vi "Teleop.vi"(10 "Match Info":T1={"Autonomous Elapsed Seconds"=0.0, "TeleOp Elapsed Seconds"=0.0, "Disabled Elapsed Seconds"=0.0, "Visited Autonomous"=FALSE, "Visited TeleOp"=FALSE, "Visited Disabled"=FALSE, "Autonomous Settings"={"Autonomous Style"=enum."Independent", "VI Refnum"=refnum}}, 11 "Call Context":T2) -> ()   [LabVIEW 2015]
doc: "This VI is called for each TeleOp packet received from the DS where the robot is not disabled. It is often used to read from the joysticks and update I/O or to update setpoints for timed control loops. It should complete and return within 20 milliseconds or it may miss DS packets."
uses:
  <vilib>/Rock Robotics/WPI/DriverStation/WPI_DriverStationDerivedRobotMode.ctl
  <vilib>/Rock Robotics/WPI/DriverStation/WPI_DriverStationMatch Info.ctl
  <vilib>/Rock Robotics/WPI/Utilities/WPI_GetSetVariantRefNum.vi
  <vilib>/Rock Robotics/Network Tables/NT Write Boolean Array.vi
  <vilib>/Rock Robotics/Network Tables/NT Write Numeric Array.vi
  <vilib>/Rock Robotics/Network Tables/NT Read Boolean.vi
  <vilib>/Rock Robotics/Network Tables/NT Read Number.vi
  <vilib>/Rock Robotics/WPI/RobotDrive/WPI_RobotDriveArcadeDrive_Standard(NoSaturation).vi
panel:
  out "Sample Slider 0":dbl(slide) scale=0.0..5.0
  out "Sample Boolean 1":bool
  out "Sample Boolean 0":bool
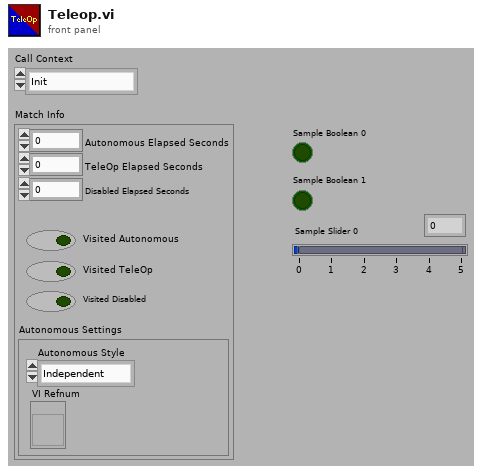
[diagram p1: front panel]
types:
  T1 = typedef "WPI_DriverStationMatch Info.ctl" = cluster{"Autonomous Elapsed Seconds":dbl, "TeleOp Elapsed Seconds":dbl, "Disabled Elapsed Seconds":dbl, "Visited Autonomous":bool, "Visited TeleOp":bool, "Visited Disabled":bool, "Autonomous Settings":cluster{"Autonomous Style":enum16{"Iterative", "Independent"}, "VI Refnum":refnum<vi>}}
  T2 = typedef "WPI_DriverStationDerivedRobotMode.ctl" = enum16{"Init", "Execute", "Stop"}
  T3 = typedef "WPI_CompressorDevRef.ctl" = cluster{"DevStatus":errorcluster, "Pneumatics Control Module":u8}
  T4 = typedef "WPI_JoystickDevRef.ctl" = cluster{"Device":T5}
  T5 = typedef "WPI_JoystickDeviceEnum.ctl" = enum16{"USB 0", "USB 1", "USB 2", "USB 3", "USB 4", "USB 5"}
  T6 = cluster{"Buttons[0]":bool, "Buttons[1]":bool, "Buttons[2]":bool, "Buttons[3]":bool, "Buttons[4]":bool, "Buttons[5]":bool, "Buttons[6]":bool, "Buttons[7]":bool, "Buttons[8]":bool}
  T7 = cluster{"Axes[0]":dbl, "Axes[1]":dbl, "Axes[2]":dbl, "Axes[3]":dbl, "Axes[4]":dbl, "Axes[5]":dbl, "Axes[6]":dbl, "Axes[7]":dbl, "Axes[8]":dbl}
  T8 = typedef "WPI_RobotDriveDevRef.ctl" = cluster{"DevStatus":errorcluster, "Motors[]":T9[], "Square Inputs":bool, "Max Output":dbl}
  T9 = typedef "WPI_MotorControlDeviceRef.ctl" = cluster{"DeviceStatus":errorcluster, "Type":T10, "PWM":cluster{"PWM Channel":T11, "DeadBand":T12}, "CAN":cluster{"Device Number":u8, "Control Mode":T13, "Semaphore":T14, "Max Vout":dbl, "TalonSRX Control Mode":T15}, "Invert":bool}
  T10 = typedef "WPI_MotorControlType.ctl" = enum16{"PWM", "CAN", "CANTalonSRX"}
  T11 = typedef "FPGA_DIOPWMChannel.ctl" = enum8{"PWM 0", "PWM 1", "PWM 2", "PWM 3", "PWM 4", "PWM 5", "PWM 6", "PWM 7", "PWM 8", "PWM 9", "PWM MXP 0", "PWM MXP 1", "PWM MXP 2", "PWM MXP 3", "PWM MXP 4", "PWM MXP 5", "PWM MXP 6", "PWM MXP 7", "PWM MXP 8", "PWM MXP 9", "Invalid"}
  T12 = typedef "WPI_PWMDeadband.ctl" = cluster{"Name":string, "maxPositivePwm":i32, "minPositivePwm":i32, "centerPwm":i32, "maxNegativePwm":i32, "minNegativePwm":i32, "angularRange":u16}
  T13 = typedef "WPI_CANJaguar_ControlMode.ctl" = enum8{"Percent VBus", "Current", "Speed", "Position", "Voltage"}
  T14 = typedef "Semaphore RefNum" = refnum<k1>
  T15 = typedef "WPI_CANTalonSRX_APIControlMode.ctl" = enum8{"Percent VBus", "Speed", "Position", "Slave", "Unchanged / Invalid", "Voltage Compensation", "Current", "Motion Profile"}
  T16 = typedef "WPI_DigitalInputDevRef.ctl" = cluster{"DevStatus":errorcluster, "DIO Channel":T17}
  T17 = typedef "FPGA_DIOChannel.ctl" = enum8{"DIO 0", "DIO 1", "DIO 2", "DIO 3", "DIO 4", "DIO 5", "DIO 6", "DIO 7", "DIO 8", "DIO 9", "DIO MXP 0", "DIO MXP 1", "DIO MXP 2", "DIO MXP 3", "DIO MXP 4", "DIO MXP 5", "DIO MXP 6", "DIO MXP 7", "DIO MXP 8", "DIO MXP 9", "DIO MXP 10", "DIO MXP 11", "DIO MXP 12", "DIO MXP 13", "DIO MXP 14", "DIO MXP 15", "Invalid"}
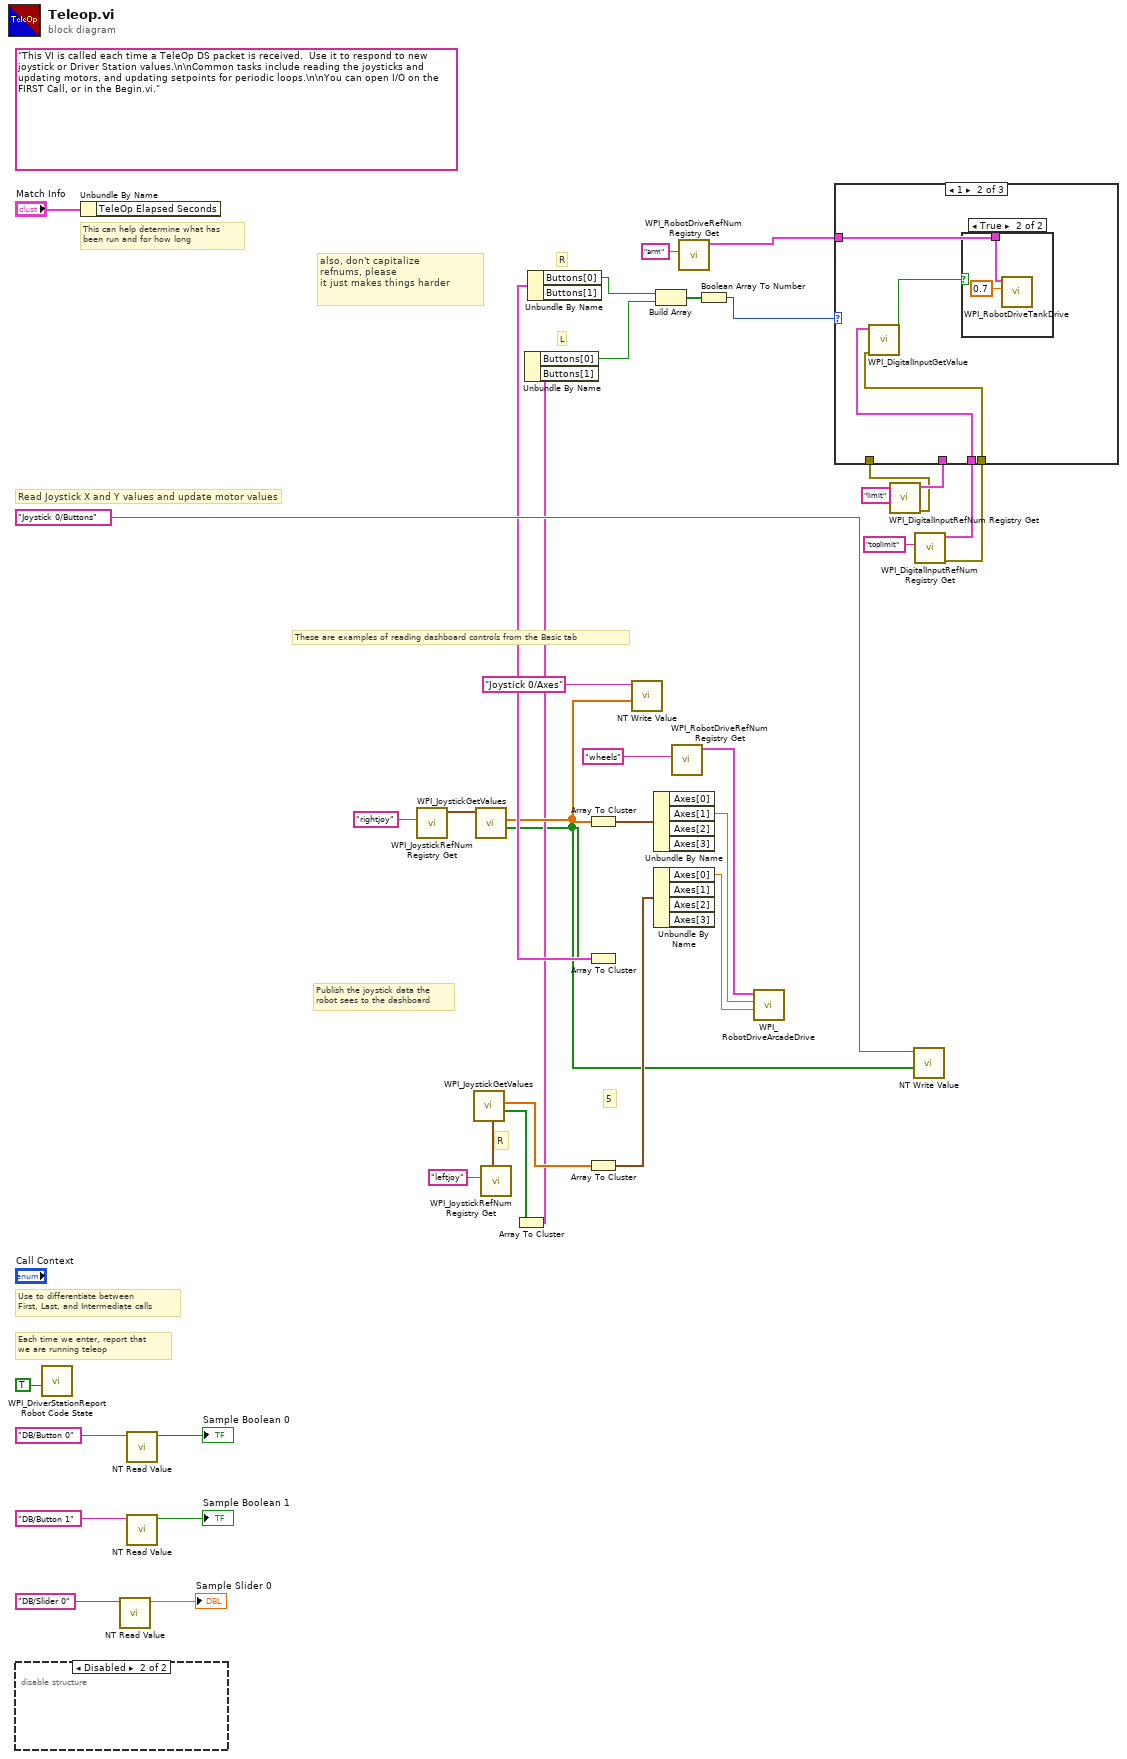
[diagram p0: block diagram]
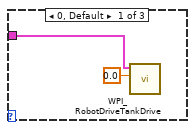
[diagram p2: hidden frame]
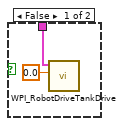
[diagram p3: hidden frame]
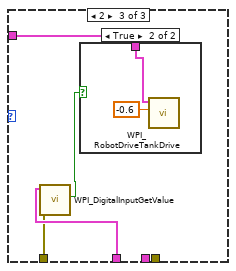
[diagram p4: hidden frame]
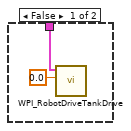
[diagram p5: hidden frame]
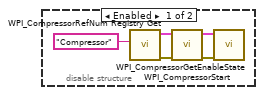
[diagram p6: hidden frame]
diagram:
  (unwired) "This VI is called each time a TeleOp DS packet is received.  Use it to respond to new joystick or Driver Station values.\n\nCommon tasks include reading the joysticks and updating motors, and updating setpoints for periodic loops.\n\nYou can open I/O on the FIRST Call, or in the Begin.vi."
  # "L"
  # "R"
  # "5"
  # "R"
  # "also, don't capitalize\nrefnums, please\nit just makes things harder"
  # "These are examples of reading dashboard controls from the Basic tab"
  # "Publish the joystick data the\nrobot sees to the dashboard"
  # "Each time we enter, report that\nwe are running teleop"
  # "Use to differentiate between\nFirst, Last, and Intermediate calls"
  # "This can help determine what has\nbeen run and for how long"
  # "Read Joystick X and Y values and update motor values"
  n1 = disable-structure shown="Disabled" {
    frame Enabled {
      n2 = call <vilib>:"WPI_CompressorRefNum Registry Get.vi"("refnum name"="Compressor") -> ("error out"=w42:errorcluster, "CompressorDevRef"=w41:T3)  [unwired: 9 in]
      n3 = call <vilib>:"WPI_CompressorStart.vi"("error in (no error)"=w42, "CompressorDevRef"=w41) -> ("error out"=w39:errorcluster, "CompressorDevRef"=w40:T3)  [unwired: 8 in]
      n4 = call <vilib>:"WPI_CompressorGetEnableState.vi"("error in (no error)"=w39, "CompressorDevRef"=w40) -> ()  [unwired: 6 in, 4 out]
    }
    frame Disabled {
    }
  }
  n5 = call <vilib>:"WPI_DriverStationReport Robot Code State.vi"("TeleOp"=TRUE ("Autonomous")) -> ()  [unwired: 10 in, 1 out]
  n6 = Unbundle By Name("Match Info") -> ()  [unwired: 1 out]
  n7 = call-poly <vilib>:"NT Read Value.vi"("Name"="DB/Slider 0" ("refnum name")) -> ("Numeric"=→"Sample Slider 0":dbl)  [unwired: 9 in, 1 out]
  n8 = call-poly <vilib>:"NT Read Value.vi"("Name"="DB/Button 0" ("refnum name")) -> ("Boolean"=→"Sample Boolean 0":bool)  [unwired: 9 in, 1 out]
  n9 = call-poly <vilib>:"NT Read Value.vi"("Name"="DB/Button 1" ("refnum name")) -> ("Boolean"=→"Sample Boolean 1":bool)  [unwired: 9 in, 1 out]
  n10 = call <vilib>:"WPI_JoystickRefNum Registry Get.vi"("refnum name"="rightjoy") -> ("JoystickDevRef"=w36:T4)  [unwired: 1 in, 9 out]
  n11 = call <vilib>:"WPI_JoystickGetValues.vi"("JoystickDevRef"=w36) -> ("Buttons"=w13:bool[], "Axes"=w21:dbl[])  [unwired: 6 in, 3 out]
  n12 = call <vilib>:"WPI_JoystickRefNum Registry Get.vi"("refnum name"="leftjoy") -> ("JoystickDevRef"=w24:T4)  [unwired: 9 in, 1 out]
  n13 = call <vilib>:"WPI_JoystickGetValues.vi"("JoystickDevRef"=w24) -> ("Buttons"=w14:bool[], "Axes"=w22:dbl[])  [unwired: 6 in, 3 out]
  n14 = Array To Cluster(array=w14) -> (cluster=w15:T6)
  n15 = Unbundle By Name(w15) -> ("Buttons[0]"=w11:bool)  [unwired: 1 out]
  n16 = Array To Cluster(array=w21) -> (cluster=w19:T7)
  n17 = Array To Cluster(array=w13) -> (cluster=w23:T6)
  n18 = Unbundle By Name(w23) -> ("Buttons[0]"=w12:bool)  [unwired: 1 out]
  n19 = Array To Cluster(array=w22) -> (cluster=w20:T7)
  n20 = call-poly <vilib>:"NT Write Value.vi"("Numeric Array"=w21, "Name"="Joystick 0/Axes") -> ()  [unwired: 9 in, 1 out]
  n21 = Unbundle By Name(w19) -> ("Axes[1]"=w17:dbl)  [unwired: 3 out]
  n22 = Unbundle By Name(w20) -> ("Axes[0]"=w16:dbl)  [unwired: 3 out]
  n23 = Build Array(w12, w11) -> (w10:bool[])
  n24 = call <vilib>:"WPI_RobotDriveRefNum Registry Get.vi"("refnum name"="wheels") -> ("RobotDriveDevRef"=w18:T8)  [unwired: 9 in, 1 out]
  n25 = call <vilib>:"WPI_RobotDriveRefNum Registry Get.vi"("refnum name"="arm") -> ("RobotDriveDevRef"=w7:T8)  [unwired: 9 in, 1 out]
  n26 = Boolean Array To Number(Boolean array=w10) -> (number=w9:u32)
  n27 = call-poly <vilib>:"WPI_RobotDriveArcadeDrive.vi"("Y axis value"=w16, "X axis value"=w17, "RobotDriveDevRef"=w18) -> ()  [unwired: 6 in, 3 out]
  n28 = call <vilib>:"WPI_DigitalInputRefNum Registry Get.vi"("refnum name"="limit") -> ("error out"=w1:errorcluster, "DigitalInputDevRef"=w2:T16)  [unwired: 9 in]
  n29 = call-poly <vilib>:"NT Write Value.vi"("Boolean Array"=w13, "Name"="Joystick 0/Buttons") -> ()  [unwired: 9 in, 1 out]
  n30 = call <vilib>:"WPI_DigitalInputRefNum Registry Get.vi"("refnum name"="toplimit") -> ("error out"=w3:errorcluster, "DigitalInputDevRef"=w4:T16)  [unwired: 9 in]
  n31 = case shown="1" w9 {
    tunnel: w7 -> [w45 w48 w56]
    tunnel: w4 -> [_ w47 _]
    tunnel: w3 -> [_ w46 _]
    tunnel: w2 -> [_ _ w55]
    tunnel: w1 -> [_ _ w54]
    frame 0, Default {
      n32 = call <vilib>:"WPI_RobotDriveTankDrive.vi"("Left axis value"=0.0, "RobotDriveDevRef"=w45) -> ()  [unwired: 7 in, 3 out]
    }
    frame 1 {
      n33 = call <vilib>:"WPI_DigitalInputGetValue.vi"("error in (no error)"=w46, "DigitalInputDevRef"=w47) -> ("Value"=w49:bool)  [unwired: 7 in, 2 out]
      n34 = case shown="True" w49 {
        tunnel: w48 -> [w50 w52]
        frame False {
          n35 = call <vilib>:"WPI_RobotDriveTankDrive.vi"("Left axis value"=0.0, "RobotDriveDevRef"=w50) -> ()  [unwired: 7 in, 3 out]
        }
        frame True {
          n36 = call <vilib>:"WPI_RobotDriveTankDrive.vi"("Left axis value"=0.7, "RobotDriveDevRef"=w52) -> ()  [unwired: 7 in, 3 out]
        }
      }
    }
    frame 2 {
      n37 = call <vilib>:"WPI_DigitalInputGetValue.vi"("error in (no error)"=w54, "DigitalInputDevRef"=w55) -> ("Value"=w57:bool)  [unwired: 7 in, 2 out]
      n38 = case shown="True" w57 {
        tunnel: w56 -> [w58 w60]
        frame False {
          n39 = call <vilib>:"WPI_RobotDriveTankDrive.vi"("Left axis value"=0.0, "RobotDriveDevRef"=w58) -> ()  [unwired: 7 in, 3 out]
        }
        frame True {
          n40 = call <vilib>:"WPI_RobotDriveTankDrive.vi"("Left axis value"=-0.6, "RobotDriveDevRef"=w60) -> ()  [unwired: 7 in, 3 out]
        }
      }
    }
  }
